vi "VISA Write String to Serial Port.vi"(2 "error in (no error)":errorcluster, 3 "String to write":string, 4 "VISA resource name":refnum<visa-resource-name>) -> (0 "error out":errorcluster, 1 "duplicate VISA resource name":refnum<visa-resource-name>)   [LabVIEW 2010]
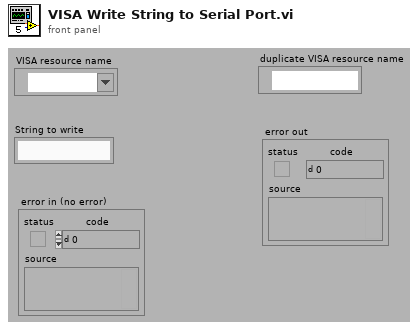
[diagram p1: front panel]
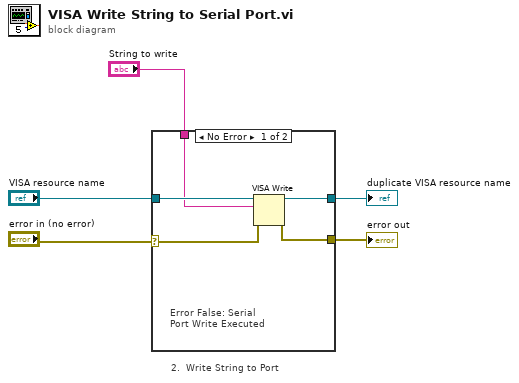
[diagram p0: block diagram]
diagram:
  # "2.  Write String to Port"
  n1 = case shown="No Error" "error in (no error)" {
    selector: "error in (no error)" -> [w9 w11]
    tunnel: "VISA resource name" -> [w10 w12]
    tunnel: [w8 w11] -> w1
    tunnel: [w7 w12] -> w2
    tunnel: "String to write" -> [w6 _]
    frame No Error {
      # "Error False: Serial\nPort Write Executed"
      n2 = VISA Write(VISA resource name=w10, write buffer=w6, error in (no error)=w9) -> (VISA resource name out=w7:refnum<visa-resource-name>, error out=w8:errorcluster)  [unwired: 1 out]
    }
    frame Error {
    }
  }
  "duplicate VISA resource name" <- w2
  "error out" <- w1
